vi "Dashboard Main.vi"() -> ()   [LabVIEW 2013]
uses:
  <vilib>/event_ctls.llb/eventvkey.ctl
  <vilib>/Rock Robotics/WPI/Dashboard/WPI_DashboardLogging Global.vi
  <vilib>/Utility/config.llb/Write Key (String).vi
  <vilib>/Utility/config.llb/Write Key (I32).vi
  <vilib>/Utility/config.llb/NI_LVConfig.lvlib
panel:
  out "Image Message":string="Timeout in Camera Communications"
  in  "Rec Mode":enum32{"Stop", "Record", "Playback"}(radio)
  in  "Dashboard Tab":T1(tab)
  in  "Camera Settings":T2={"Frame Rate"=30, "Compression"=30, "Size"=1} {"Frame Rate" scale=1.0..30.0; "Size" items=["640x480", "320x240", "160x120"]}
  out "MotorSliders R":cluster{"MotorSlide1":dbl, "MotorSlide2":dbl} {"MotorSlide2" scale=-1.0..1.0 scale format="%#_2e"; "MotorSlide1" scale=-1.0..1.0 scale format="%#_2e"}
  out "MotorChart R":cluster{"Numeric":dbl, "Numeric":dbl}(graph)
  out "MotorSliders L":T3 {"MotorSlide4 2" scale=0.0..14.0 scale format="%#_2e"; "MotorSlide2" scale=-1.0..1.0 scale format="%#_2e"; "MotorSlide1" scale=-1.0..1.0 scale format="%#_2e"}
  out "MotorChart L":T4(graph)
  out "JS1 Z":dbl(slide) scale=-1.0..1.0 scale format="%#_2e"
  out "Joystick 1":cluster{"X":dbl, "Y":dbl}[](graph)
  out "JS Buttons 1":T5
  out "JS2 Z":dbl(slide) scale=-1.0..1.0 scale format="%#_2e"
  out "Joystick 2":cluster{"X":dbl, "Y":dbl}[](graph)
  out "JS Buttons 2":T5
  out "Mode":T6(ring)=enum."Auto Disabled"
  out "Camera IP":string
  in  "DB Camera Config":bool
  out "fps":dbl format="%#.1g"
  out "Mbps":dbl format="%#.1g"
  out "Mbps 2":bool
  out "LED 1":bool
  in  "Experimental Features":bool
  in  "Camera Light":bool
  out "Shot Duration":dbl
  out "Shooting":bool
  in  "Fake LS":bool
  out "Light":dbl
  in  "Zero Encoders":bool
  out "Right Encoder":dbl
  out "Left Encoder":dbl
  out "Ultrasonic":dbl(slide) scale=0.0..14.0
  out "Pickup Solenoid Reverse":bool
  out "Pickup Solenoid Forward":bool
  out "Shooter Solenoid":bool
  out "Robot Code Version":string
  in  "Auto Routine":dbl
  in  "Shoot Distance":dbl
  in  "Distance from Tape":dbl
  out "Vision Display":T7(plugin-control)
  in  "Vision Processing":bool
  in  "Annotation":bool=TRUE
  in  "Retroreflective Processing":bool=TRUE
  in  "Team Color Processing":bool=TRUE
  out "Number of Particles":i32
  in  "Threshold Values":T8(array[cluster])
  in  "Introduce Photo":bool
  in  "Picture Input":path
  in  "Test Slider":dbl(slide) scale=0.0..100.0 scale format="%#_3g"
  in  "On/Off":bool caption="Solenoid"
  in  "Test Name":u16(ring) items=["Select the test to run...", "Example Test", "-------------------------------", "List of tests is built in robot code.", "Replace with your own automated tests."]
  in  "Test Tree":string(tree)
  in  "Motor":cluster{"Value":dbl, "Enable":bool} {"Value" scale=-1.0..1.0 scale format="%#_3g"}
  out "Progress":T9 {"Test Progress" scale=0.0..100.0}
  in  "Rev/Fwd":cluster{"Forward":bool, "Reverse":bool}
  in  "Test Ring":u16(ring) items=["Auto", "Fixed indoor", "Fixed outdoor 1", "Fixed outdoor 2", "Fixed fluorescent 1", "Fixed fluorescent 2", "Hold current"]
  in  "Listbox":i32(listbox)
  out "Tree":string(tree)
  out "Camera Image":T7(plugin-control)
  in  "Enable":bool
  # "Left"
  # "Front"
  # "Right"
  # "Battery"
  # "Set to 0 for none\nSet to 1 for Auto 1"
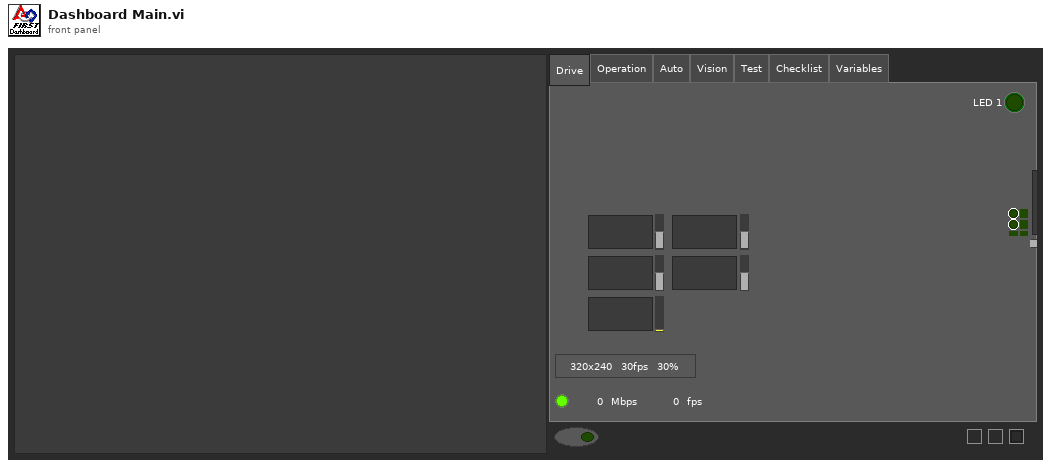
[diagram p1: front panel]
types:
  T1 = enum32{"Drive", "Operation", "Auto", "Vision", "Test", "Checklist", "Variables"}
  T2 = cluster{"Frame Rate":i32, "Compression":i32, "Size":u16}
  T3 = cluster{"MotorSlide1":dbl, "MotorSlide2":dbl, "MotorSlide4 2":dbl}
  T4 = cluster{"Numeric":dbl, "Numeric":dbl, "Battery":sgl}
  T5 = cluster{bool, bool, bool, bool, bool, bool, bool, bool, bool, bool, bool, bool}
  T6 = enum8{"Tele-Op Disabled", "Tele-Op Enabled", "Auto Disabled", "Auto Enabled", "Test Disabled", "Test Enabled", ""}
  T7 = typedef "IMAQ Image.ctl" = refnum<image>
  T8 = cluster{"Blue or Luma or Val or Inten Range":cluster{"Lower value":i32, "Upper value":i32}, "Red or Hue Range":cluster{"Lower value":i32, "Upper value":i32}, "Green or Sat Range":cluster{"Lower value":i32, "Upper value":i32}}[]
  T9 = cluster{"Test Progress":u8, "Test Progress Text":string}
  T10 = enum32{"Drive", "Operation", "Auto", "Test", "Checklist", "Variables"}
  T11 = typedef "Image Type" = u32
  T12 = cluster{"Digital Inputs":bool[], "Digital Outputs":bool[]}
  T13 = cluster{"Competition mode":bool, "Robot Link":bool, "Autonomous":bool, "Enabled":bool, "E-Stop":bool, "Simulated":bool, "TestMode":bool, "Docked Window":bool}
  T14 = cluster{"Boolean Array[0]":bool, "Boolean Array[1]":bool, "Boolean Array[2]":bool, "Boolean Array[3]":bool, "Boolean Array[4]":bool, "Boolean Array[5]":bool, "Boolean Array[6]":bool, "Boolean Array[7]":bool, "Boolean Array[8]":bool, "Boolean Array[9]":bool, "Boolean Array[10]":bool, "Boolean Array[11]":bool}
  T15 = typedef "NI_LVConfig.lvlib/Config Data RefNum.ctl" = refnum<k1>
  T16 = typedef "eventvkey.ctl" = enum16{"ASCII", "Enter", "Return", "Shift", "Ctrl", "Alt", "Cmd", "Opt", "Caps", "NumLock", "Clear", "Break", "Up", "Down", "Left", "Right", "Insert", "Delete", "Home", "End", "PageUp", "PageDown", "Escape", "Help", "Pause", "ScrollLock", "F1", "F2", "F3", "F4", "F5", "F6", "F7", "F8", "F9", "F10", "F11", "F12", "F13", "F14", "F15", "F16", "F17", "F18", "F19", "F20", "F21", "F22", "F23", "F24", "Play", "VolumeUp", "VolumeDown", "Mute", "Two Byte Char"}
  T17 = cluster{"Image Size":bool, "Image Type":bool, "Pixel Value":bool, "ROI Information":bool, "Zoom Factor":bool}
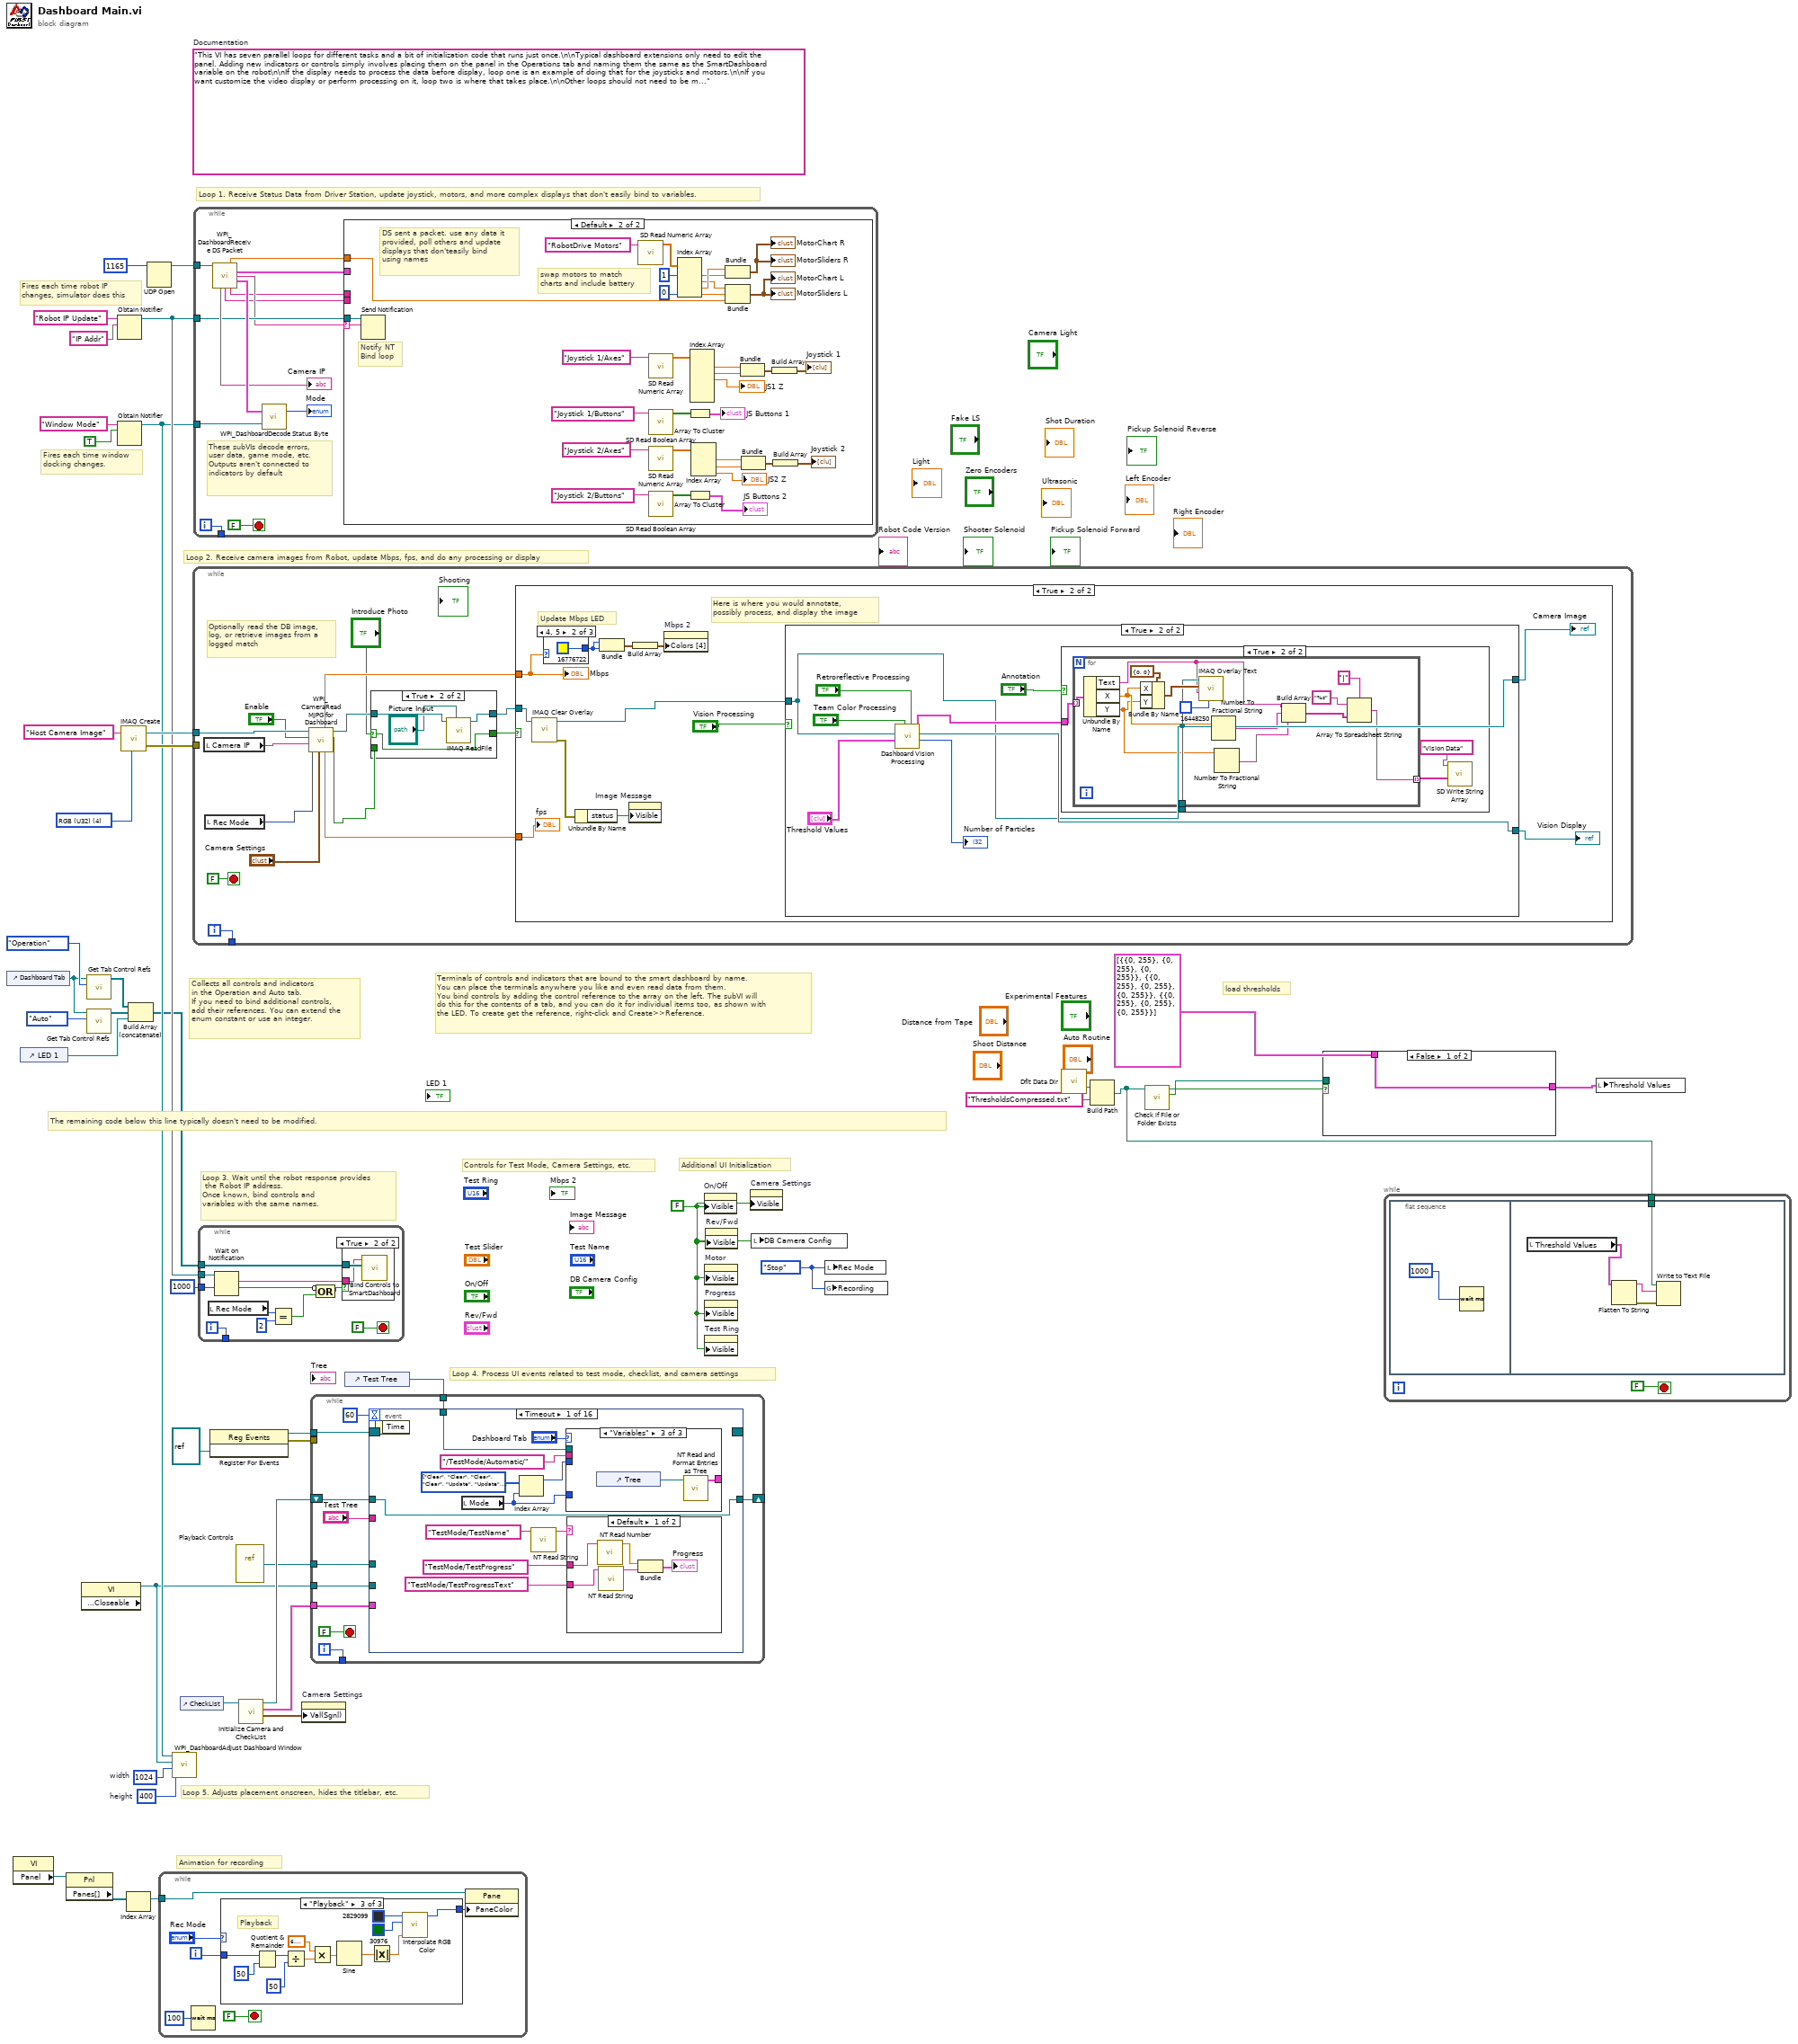
[diagram p0: block diagram]
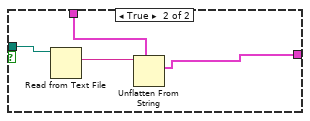
[diagram p2: hidden frame]
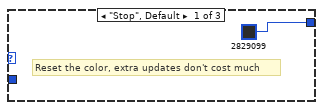
[diagram p3: hidden frame]
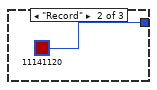
[diagram p4: hidden frame]
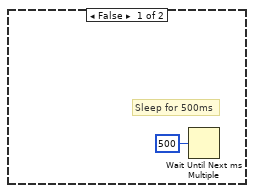
[diagram p7: hidden frame]
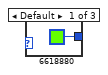
[diagram p10: hidden frame]
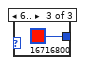
[diagram p11: hidden frame]
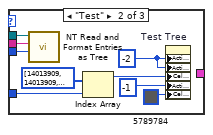
[diagram p13: hidden frame]
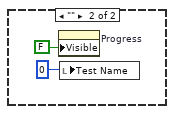
[diagram p14: hidden frame]
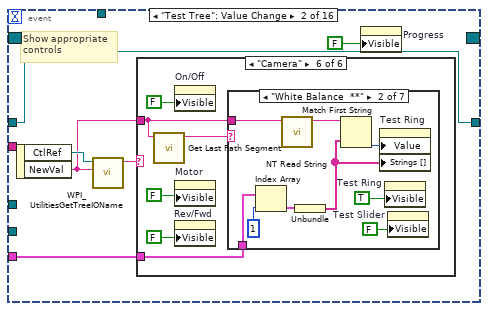
[diagram p15: hidden frame]
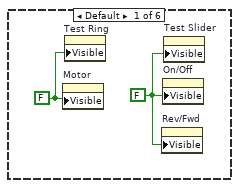
[diagram p16: hidden frame]
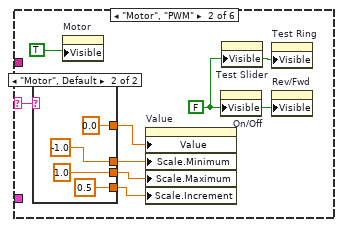
[diagram p17: hidden frame]
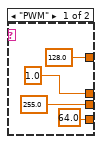
[diagram p18: hidden frame]
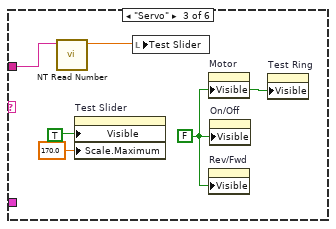
[diagram p19: hidden frame]
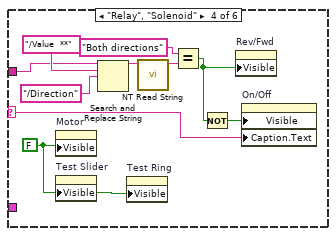
[diagram p20: hidden frame]
diagram:
  w15 = enum32{"Stop", "Record", "Playback"}."Stop" ("Rec Mode")
  w18 = 400  # height
  w19 = 1024  # width
  w32 = FALSE ("Visible")
  (unwired) "This VI has seven parallel loops for different tasks and a bit of initialization code that runs just once.\n\nTypical dashboard extensions only need to edit the panel. Adding new indicators or controls simply involves placing them on the panel in the Operations tab and naming them the same as the SmartDashboard variable on the robot\n\nIf the display needs to process the data before display, loop one is an example of doing that for the joysticks and motors.\n\nIf you want customize the video display or perform processing on it, loop two is where that takes place.\n\nOther loops should not need to be modified. They are pretty standard, and document the task they perform."  # Documentation
  w42 = T11 4 items=["Grayscale (U8)", "Grayscale (I16)", "Grayscale (SGL)", "Complex (CSG)", "RGB (U32)", "HSL (U32)", "RGB (U64)"] ("Image Type")
  # "load thresholds"
  # "Controls for Test Mode, Camera Settings, etc."
  # "Additional UI Initialization"
  # "Animation for recording"
  # "Fires each time robot IP\nchanges, simulator does this"
  # "Fires each time window\ndocking changes."
  # "Collects all controls and indicators\nin the Operation and Auto tab.\nIf you need to bind additional controls,\nadd their references. You can extend the\nenum constant or use an integer."
  # "The remaining code below this line typically doesn't need to be modified."
  # "Loop 4. Process UI events related to test mode, checklist, and camera settings"
  # "Terminals of controls and indicators that are bound to the smart dashboard by name.\nYou can place the terminals anywhere you like and even read data from them.\nYou bind controls by adding the control reference to the array on the left. The subVI will\ndo this for the contents of a tab, and you can do it for individual items too, as shown with\nthe LED. To create get the reference, right-click and Create>>Reference."
  # "Loop 3. Wait until the robot response provides\n the Robot IP address.\nOnce known, bind controls and\nvariables with the same names."
  # "Loop 5. Adjusts placement onscreen, hides the titlebar, etc."
  # "Loop 1. Receive Status Data from Driver Station, update joystick, motors, and more complex displays that don't easily bind to variables."
  # "Loop 2. Receive camera images from Robot, update Mbps, fps, and do any processing or display"
  n1 = control-ref of="Dashboard Tab"() -> (w13:refnum<vi>)
  n2 = property class="VI"() -> ("Panel"=w26:refnum<vi>)  [unwired: 2 in, 2 out]
  n3 = control-ref of="LED 1"() -> (w8:refnum<vi>)
  n4 = property class="Pnl"(reference=w26) -> ("Panes[]"=w27:refnum<vi>[])  [unwired: 1 in, 2 out]
  n5 = property class="VI" props=["Front Panel.Closeable"]() -> (reference out=w14:refnum<vi>)  [unwired: 2 in, 2 out]
  n6 = call <vilib>:"Get Tab Control Refs.vi"("Page Index"=T10."Operation" ("Dashboard Tab"), "TabControl in"=w13) -> ("ControlsOnPage"=w11:refnum<vi>[])  [unwired: 9 in]
  n7 = call <vilib>:"Get Tab Control Refs.vi"("Page Index"=T10."Auto" ("Dashboard Tab"), "TabControl in"=w13) -> ("ControlsOnPage"=w12:refnum<vi>[])  [unwired: 9 in]
  n8 = Obtain Notifier(name (unnamed)="Robot IP Update", notification data type="IP Addr" ("name (unnamed)")) -> (notifier out=w36:refnum<notifier>)  [unwired: 2 in, 2 out]
  n9 = Obtain Notifier(name (unnamed)="Window Mode", notification data type=TRUE) -> (notifier out=w17:refnum<notifier>)  [unwired: 2 in, 2 out]
  n10 = call "IMAQ Create"("Image Name"="Host Camera Image", "Image Type"=w42) -> ("New Image"=w40:T7, "error out"=w39:errorcluster)  [unwired: 2 in, 1 out]
  n11 = Index Array(array=w27) -> (element=w25:refnum<vi>)  [unwired: 1 in]
  n12 = Build Array (concatenate)(w11, w12, w8) -> (w10:refnum<vi>[])
  n13 = UDP Open(11:u16 1165 ("port")) -> (port=w43:refnum<k16>)  [unwired: 2 in, 4 out]
  n14 = while {
    tunnel: w25 -> [w46]
    i -> [w49]
    stop <- FALSE stop-if-true
    n15 = Wait (ms)(milliseconds to wait=u32 100) -> ()  [unwired: 1 out]
    n16 = case shown="\"Playback\"" "Rec Mode" {
      tunnel: w49 -> [_ _ w64]
      tunnel: [u32 2829099 ("Base Color") u32 11141120 ("Target Color") w53] -> w45
      frame "Stop", Default {
        # "Reset the color, extra updates don't cost much"
      }
      frame "Record" {
      }
      frame "Playback" {
        # "Playback"
        n17 = Quotient & Remainder(x=w64, y=u32 50 ("milliseconds to wait")) -> (x-y*floor(x/y)=w60:u32)  [unwired: 1 out]
        n18 = Divide(x=w60, y=u32 50 ("milliseconds to wait")) -> (x/y=w57:dbl)
        n19 = Multiply(x=6.283185307179586, y=w57) -> (x*y=w62:dbl)
        n20 = Sine(x=w62) -> (sin(x)=w61:dbl)
        n21 = Absolute Value(x=w61) -> (abs(x)=w54:dbl)
        n22 = call "Interpolate RGB Color.vi"("Proportion"=w54, "Target Color"=u32 30976, "Base Color"=u32 2829099) -> ("Result Color"=w53:u32)  [unwired: 8 in]
      }
    }
    n23 = property class="Pane"(reference=w46, "PaneColor"=w45) -> ()  [unwired: 1 in, 2 out]
  }
  n24 = call <vilib>:"WPI_DashboardAdjust Dashboard Window.vi"("height"=w18, "width"=w19, "reference in"=w14, "Notifier in"=w17) -> ()  [unwired: 8 in]
  n25 = control-ref of="CheckList"() -> (w16:refnum<vi>)
  n26 = while {
    tunnel: w40 -> [w76]
    tunnel: w39 -> [_]
    tunnel: [w77] -> _
    i -> [w77]
    stop <- FALSE stop-if-true
    # "Optionally read the DB image,\nlog, or retrieve images from a\nlogged match"
    n27 = local read "Camera IP"() -> (w71:string)
    n28 = local read "Rec Mode"() -> (w70:enum32{"Stop", "Record", "Playback"})
    n29 = call <vilib>:"WPI_CameraRead MJPG for Dashboard.vi"("Camera Settings"="Camera Settings", "Rec Mode"=w70, "Camera IP"=w71, "Enable"="Enable", "Refnum in"=w76) -> ("Active"=w66:bool, "Refnum out"=w69:T7, "FPS"=w74:dbl, "Bandwidth (Mbps)"=w73:dbl)  [unwired: 3 in]
    n30 = case shown="True" "Introduce Photo" {
      selector: "Introduce Photo" -> [_ w81]
      tunnel: w69 -> [w80 w84]
      tunnel: [w80 w83] -> w68
      tunnel: w66 -> [w79 _]
      tunnel: [w79 w81] -> w65
      frame False {
      }
      frame True {
        n31 = call "IMAQ ReadFile"("File Path"="Picture Input", "Image"=w84) -> ("Image Out"=w83:T7)  [unwired: 5 in, 4 out]
      }
    }
    n32 = case shown="True" w65 {
      tunnel: w73 -> [_ w92]
      tunnel: w74 -> [_ w91]
      tunnel: w68 -> [_ w87]
      frame False {
        # "Sleep for 500ms"
        n33 = Wait Until Next ms Multiple(millisecond multiple=u32 500) -> ()  [unwired: 1 out]
      }
      frame True {
        # "Here is where you would annotate,\npossibly process, and display the image"
        # "Update Mbps LED"
        n34 = call "IMAQ Clear Overlay"("Image"=w87) -> ("error out"=w96:errorcluster, "Image Out"=w89:T7)  [unwired: 2 in, 7 out]
        n35 = case shown="4, 5" w92 {
          tunnel: [u32 6618880 ("Color Box") u32 16776722 ("Color Box") u32 16716800 ("Color Box")] -> w93
          frame Default {
          }
          frame 4, 5 {
          }
          frame 6.. {
          }
        }
        n36 = Unbundle By Name(w96) -> ("status"=w97:bool)
        n37 = Bundle("Color Box"=w93, "Color Box"=w93) -> (w95:cluster{"Color Box":u32, "Color Box":u32})  [unwired: 1 out]
        n38 = property on="Image Message" class="Str"("Visible"=w97) -> ()  [unwired: 2 in, 2 out]
        n39 = Build Array(w95) -> (w94:cluster{"Color Box":u32, "Color Box":u32}[])
        n40 = property on="Mbps 2" class="Bool (strict)"("Colors [4]"=w94) -> ()  [unwired: 2 in, 2 out]
        n41 = case shown="True" "Vision Processing" {
          tunnel: w89 -> [w98 w100]
          tunnel: [w98 w106] -> w86
          tunnel: [w98 w100] -> w88
          frame False {
          }
          frame True {
            n42 = call "Dashboard Vision Processing.vi"("Retroreflective Processing"="Retroreflective Processing", "Team Color Processing"="Team Color Processing", "Threshold Values"="Threshold Values", "Camera Image"=w100) -> ("Number of Particles"=→"Number of Particles":i32, "Retro Image"=w106:T7, "Annotations"=w101:cluster{"Text":string, "X":dbl, "Y":dbl}[])  [unwired: 4 in, 1 out]
            n43 = case shown="True" "Annotation" {
              tunnel: w101 -> [_ w110]
              tunnel: w100 -> [_ w109]
              frame False {
              }
              frame True {
                n44 = for {
                  tunnel: w110 -> [w124] mode=indexing
                  tunnel: w109 -> [w121]
                  tunnel: [w111] -> w108 mode=indexing
                  n45 = Unbundle By Name(w124) -> ("Text"=w117:string, "X"=w120:dbl, "Y"=w119:dbl)
                  n46 = Bundle By Name(cluster=cluster{"X":i32, "Y":i32} {"X"=0, "Y"=0} ("Origin"), "X"=w120, "Y"=w119) -> (w122:cluster{"X":i32, "Y":i32})
                  n47 = call "IMAQ Overlay Text"("Text Color (black)"=u32 16448250, "String"=w117, "Origin"=w122, "Image"=w121) -> ()  [unwired: 6 in, 2 out]
                  n48 = Number To Fractional String(number=w120) -> (F-format string=w116:string)  [unwired: 3 in]
                  n49 = Number To Fractional String(number=w119) -> (F-format string=w115:string)  [unwired: 3 in]
                  n50 = Build Array(w117, w116, w115) -> (w114:string[])
                  n51 = Array To Spreadsheet String(delimiter (Tab)="|", array=w114, 3:"%s") -> (spreadsheet string=w111:string)
                }
                n52 = call <vilib>:"SD Write String Array.vi"("String Array"=w108, "Name"="Vision Data") -> ()  [unwired: 8 in, 2 out]
              }
            }
          }
        }
        "Camera Image" <- w88
        "Vision Display" <- w86
        "Mbps" <- w92
        "fps" <- w91
      }
    }
  }
  n53 = while {
    tunnel: w43 -> [w138]
    tunnel: w36 -> [w133]
    tunnel: w17 -> [w137]
    tunnel: [w134] -> _
    i -> [w134]
    stop <- FALSE stop-if-true
    # "These subVIs decode errors, user data, game mode, etc.\nOutputs aren't connected to indicators by default"
    n54 = call <vilib>:"WPI_DashboardReceive DS Packet.vi"("Recv Socket"=w138) -> ("Battery"=w128:sgl, "Driver Station"=w129:T12, "Robot IP Address"=w132:string, "Status"=w139:T13, "Camera IP Address"=→"Camera IP":string, "Low Priority User Data"=w131:string, "High Priority User Data"=w130:string)  [unwired: 1 in, 7 out]
    n55 = call <vilib>:"WPI_DashboardDecode Status Byte.vi"("Window Mode Notifier"=w137, "Status"=w139) -> ("Mode"=→"Mode":T6)  [unwired: 1 out]
    n56 = case shown="Default" w132 {
      selector: w132 -> [_ w151]
      tunnel: w133 -> [_ w152]
      tunnel: w131 -> [_ _]
      tunnel: w130 -> [_ _]
      tunnel: w129 -> [_ _]
      tunnel: w128 -> [_ w150]
      frame "0.0.0.0" {
        # "DS not sending packets, or no robot exists yet.\nDon't poll the variables"
      }
      frame Default {
        # "Notify NT\nBind loop"
        # "DS sent a packet. use any data it\nprovided, poll others and update\ndisplays that don'teasily bind\nusing names"
        # "swap motors to match\ncharts and include battery"
        n57 = Send Notification(notification=w151, notifier=w152) -> ()  [unwired: 1 in, 2 out]
        n58 = call <vilib>:"SD Read Numeric Array.vi"("Name"="RobotDrive Motors") -> ("Numeric Array"=w149:dbl[])  [unwired: 8 in, 2 out]
        n59 = call <vilib>:"SD Read Numeric Array.vi"("Name"="Joystick 1/Axes") -> ("Numeric Array"=w168:dbl[])  [unwired: 8 in, 2 out]
        n60 = call <vilib>:"SD Read Boolean Array.vi"("Name"="Joystick 1/Buttons") -> ("Boolean Array"=w170:bool[])  [unwired: 8 in, 2 out]
        n61 = call <vilib>:"SD Read Numeric Array.vi"("Name"="Joystick 2/Axes") -> ("Numeric Array"=w162:dbl[])  [unwired: 8 in, 2 out]
        n62 = call <vilib>:"SD Read Boolean Array.vi"("Name"="Joystick 2/Buttons") -> ("Boolean Array"=w161:bool[])  [unwired: 8 in, 2 out]
        n63 = Index Array(array=w149, index #1=1, index #4=0) -> (element #1=w145:dbl, element #2=w144:dbl, element #3=w146:dbl, element #4=w141:dbl)  [unwired: 2 in]
        n64 = Array To Cluster(array=w170) -> (cluster=→"JS Buttons 1":T14)
        n65 = Array To Cluster(array=w161) -> (cluster=→"JS Buttons 2":T14)
        n66 = Index Array(array=w168) -> (element #1=w165:dbl, element #2=w166:dbl, element #3=→"JS1 Z":dbl)  [unwired: 6 in, 3 out]
        n67 = Index Array(array=w162) -> (element #1=w157:dbl, element #2=w156:dbl, element #3=→"JS2 Z":dbl)  [unwired: 3 in]
        n68 = Bundle("Numeric"=w146, "Numeric"=w145) -> (→"MotorChart R" →"MotorSliders R":cluster{"Numeric":dbl, "Numeric":dbl})  [unwired: 1 in]
        n69 = Bundle("Numeric"=w144, "Numeric"=w141, "Battery"=w150) -> (→"MotorChart L" →"MotorSliders L":T4)  [unwired: 1 in]
        n70 = Bundle("Numeric"=w165, "Numeric"=w166) -> (w164:cluster{"Numeric":dbl, "Numeric":dbl})  [unwired: 1 in]
        n71 = Bundle("Numeric"=w157, "Numeric"=w156) -> (w158:cluster{"Numeric":dbl, "Numeric":dbl})  [unwired: 1 in]
        n72 = Build Array(w164) -> (→"Joystick 1":cluster{"Numeric":dbl, "Numeric":dbl}[])
        n73 = Build Array(w158) -> (→"Joystick 2":cluster{"Numeric":dbl, "Numeric":dbl}[])
      }
    }
  }
  n74 = while {
    tunnel: w10 -> [w184]
    tunnel: w36 -> [w182]
    tunnel: [w180] -> _
    tunnel: u32 1000 ("milliseconds to wait") -> [w179]
    i -> [w180]
    stop <- FALSE stop-if-true
    n75 = local read "Rec Mode"() -> (w175:enum32{"Stop", "Record", "Playback"})
    n76 = Wait on Notification(notifier=w182, timeout in ms (-1)=w179) -> (notification=w181:string, timed out?=w177:bool)  [unwired: 2 in, 2 out]
    n77 = Equal?(x=w175, y=u16 2 ("Rec Mode")) -> (x = y?=w176:bool)
    n78 = Compound Arithmetic op=OR(invert w177, w176) -> (w178:bool)
    n79 = case shown="True" w178 {
      tunnel: w184 -> [_ w186]
      tunnel: w181 -> [_ w185]
      frame False {
      }
      frame True {
        n80 = call <vilib>:"Bind Controls to SmartDashboard.vi"("Bound Control Refs"=w186, "Server IP Address"=w185) -> ()  [unwired: 10 in]
      }
    }
  }
  n81 = register-events(refnum<vi> refnum) -> (reference out=w23:refnum<event-registration>, error out=w22:errorcluster)  [unwired: 2 in]
  n82 = vi-ref "Playback Controls.vi"() -> (w24:refnum<vi>)
  n83 = call "Initialize Camera and CheckList.vi"("ListBox in"=w16) -> ("Cluster"=w30:cluster{"value":i32, "value":i32, "index":i32}, "Array"=w31:cluster{string[]}[], "File Refnum"=w29:T15)  [unwired: 8 in]
  n84 = property on="Camera Settings" class="Clust (strict)"("Val(Sgnl)"=w30) -> ()  [unwired: 2 in, 2 out]
  n85 = control-ref of="Test Tree"() -> (w28:refnum<vi>)
  n86 = while {
    tunnel: w31 -> [w194]
    shift-right: [w193] -> _
    shift-left: w29 -> [w192]
    tunnel: [w191] -> _
    tunnel: w28 -> [w190]
    tunnel: w24 -> [w189]
    tunnel: w23 -> [w188]
    tunnel: w22 -> [_]
    tunnel: w14 -> [w187]
    i -> [w191]
    stop <- FALSE stop-if-true
    n87 = event shown="[0] Timeout" {
      selector: w188 -> [_ _ _ _ _ _ _ _ _ _ _ _ _ _ _ _]
      dyn-events: [_ _ _ _ _ _ _ _ _ _ _ _ _ w432 _ _] -> _
      timeout: u32 60 ("milliseconds to wait") -> [_ _ _ _ _ _ _ _ _ _ _ _ _ _ _ _]
      tunnel: w190 -> [w204 _ _ _ _ _ _ _ _ _ _ _ _ _ _ _]
      tunnel: "Test Tree" -> [_ _ _ _ _ _ _ _ w401 w409 w411 w415 w423 _ _ _]
      tunnel: w194 -> [_ w228 _ _ _ _ w365 w395 _ _ _ _ _ _ _ _]
      tunnel: [w198 w227 w326 w331 w339 w351 w364 w388 w400 w407 w410 w414 w422 w434 w448 w449] -> w193
      tunnel: w192 -> [w198 w227 w326 w331 w339 w351 w363 w388 w400 w407 w410 w414 w422 w434 w448 w449]
      tunnel: w189 -> [_ _ _ _ _ _ _ _ _ _ _ _ _ w435 _ w452]
      tunnel: w187 -> [_ _ _ _ _ _ _ _ _ _ _ _ _ w430 _ _]
      event Timeout {
        w203 = enum16{"Update", "Clear"}[] [enum."Clear", enum."Clear", enum."Clear", enum."Clear", enum."Update", enum."Update", enum."Clear"] items=["Update", "Clear"]
        n88 = event-data() -> ()  [unwired: 1 in, 1 out]
        n89 = local read "Mode"() -> (w201:T6)
        n90 = Index Array(array=w203, index=w201) -> (element=w202:enum16{"Update", "Clear"})
        n91 = call <vilib>:"NT Read String.vi"("Name"="TestMode/TestName") -> ("String"=w207:string)  [unwired: 9 in, 1 out]
        n92 = case shown="\"Variables\"" "Dashboard Tab" {
          tunnel: w204 -> [_ w217 _]
          tunnel: "/TestMode/Automatic/" ("Name Pattern") -> [_ w216 _]
          tunnel: w202 -> [_ w215 _]
          tunnel: w201 -> [_ w213 _]
          tunnel: [_ _ w219] -> _
          frame "Operation", Default {
          }
          frame "Test" {
            w212 = -2 ("Active Item:Row Number")
            n93 = call <vilib>:"NT Read and Format Entries as Tree.vi"("Operation"=w215, "Name Pattern"=w216, "Tree Refnum"=w217) -> ()  [unwired: 7 in, 2 out]
            n94 = Index Array(array=u32[] [14013909, 14013909, 14013909, 14013909, 14013909, 16777215, 14013909], index=w213) -> (element=w211:u32)
            n95 = property on="Test Tree" class="Tree (strict)"("Active Item Row Number"=w212, "ActiveColNum"=w212, "CellBG"=w211, "Active Item Row Number"=-1 ("Active Item:Row Number"), "CellBG"=u32 5789784 ("Color Box")) -> ()  [unwired: 2 in, 2 out]
          }
          frame "Variables" {
            n96 = control-ref of="Tree"() -> (w218:refnum<vi>)
            n97 = call <vilib>:"NT Read and Format Entries as Tree.vi"("Tree Refnum"=w218) -> ("Formatted Strings"=w219:cluster{"Name":string, "Value":string}[])  [unwired: 9 in, 1 out]
          }
        }
        n98 = case shown="Default" w207 {
          tunnel: "TestMode/TestProgress" ("Name") -> [w221 _]
          tunnel: "TestMode/TestProgressText" ("Name") -> [w220 _]
          frame Default {
            n99 = call <vilib>:"NT Read Number.vi"("Name"=w221) -> ("Numeric"=w222:dbl)  [unwired: 9 in, 1 out]
            n100 = call <vilib>:"NT Read String.vi"("Name"=w220) -> ("String"=w223:string)  [unwired: 9 in, 1 out]
            n101 = Bundle("Numeric"=w222, "String"=w223) -> (→"Progress":cluster{"Numeric":dbl, "String":string})  [unwired: 1 in]
          }
          frame "" {
            n102 = property on="Progress" class="Clust (strict)"("Visible"=FALSE) -> ()  [unwired: 2 in, 2 out]
            n103 = local write "Test Name"(u16 0) -> ()
          }
        }
      }
      event "Test Tree": Value Change {
        # "Show appropriate\ncontrols"
        n104 = event-data() -> ("CtlRef"=w231:refnum<vi>, "NewVal"=w229:string)  [unwired: 1 in]
        n105 = call <vilib>:"WPI_UtilitiesGetTreeIOName.vi"("NewVal"=w229, "TreeControl in"=w231) -> ("I/O Name"=w232:string)  [unwired: 9 in]
        n106 = case shown="\"Camera\"" w232 {
          selector: w232 -> [_ w239 _ w257 w266 _]
          tunnel: w229 -> [_ _ w254 w256 _ w273]
          tunnel: w228 -> [_ _ _ _ _ w272]
          frame Default {
            w234 = FALSE ("Visible")
            w233 = FALSE ("Visible")
            n107 = property on="Motor" class="Clust (strict)"("Visible"=w233) -> ()  [unwired: 2 in, 2 out]
            n108 = property on="Test Ring" class="Ring (strict)"("Visible"=w233) -> ()  [unwired: 2 in, 2 out]
            n109 = property on="Rev/Fwd" class="Clust (strict)"("Visible"=w234) -> ()  [unwired: 2 in, 2 out]
            n110 = property on="On/Off" class="Bool (strict)"("Visible"=w234) -> ()  [unwired: 2 in, 2 out]
            n111 = property on="Test Slider" class="Slide (strict)"("Visible"=w234) -> ()  [unwired: 2 in, 2 out]
          }
          frame "Motor", "PWM" {
            w240 = FALSE ("Visible")
            n112 = case shown="\"Motor\", Default" w239 {
              tunnel: [1.0 ("Value") -1.0 ("Value")] -> w238
              tunnel: [255.0 ("Value") 1.0 ("Value")] -> w237
              tunnel: [128.0 ("Value") 0.0 ("Value")] -> w236
              tunnel: [64.0 ("Value") 0.5 ("Value")] -> w235
              frame "PWM" {
              }
              frame "Motor", Default {
              }
            }
            n113 = property on="Motor" class="Clust (strict)"("Visible"=TRUE) -> ()  [unwired: 2 in, 2 out]
            n114 = property on="Value" class="Slide (strict)"("Value"=w236, "Scale.Minimum"=w238, "Scale.Maximum"=w237, "Scale.Increment"=w235) -> ()  [unwired: 2 in, 2 out]
            n115 = property on="On/Off" class="Bool (strict)"("Visible"=w240) -> ()  [unwired: 2 in, 2 out]
            n116 = property on="Test Slider" class="Slide (strict)"("Visible"=w240) -> ()  [unwired: 2 in, 2 out]
            n117 = property on="Test Ring" class="Ring (strict)"("Visible"=w240) -> ()  [unwired: 2 in, 2 out]
            n118 = property on="Rev/Fwd" class="Clust (strict)"("Visible"=w240) -> ()  [unwired: 2 in, 2 out]
          }
          frame "Servo" {
            w252 = FALSE ("Visible")
            n119 = call <vilib>:"NT Read Number.vi"("Name"=w254) -> ("Numeric"=w253:dbl)  [unwired: 9 in, 1 out]
            n120 = property on="Test Slider" class="Slide (strict)"("Visible"=TRUE, "Scale.Maximum"=170.0 ("Scale.Range:Maximum")) -> ()  [unwired: 2 in, 2 out]
            n121 = local write "Test Slider"(w253) -> ()
            n122 = property on="Motor" class="Clust (strict)"("Visible"=w252) -> ()  [unwired: 2 in, 2 out]
            n123 = property on="Rev/Fwd" class="Clust (strict)"("Visible"=w252) -> ()  [unwired: 2 in, 2 out]
            n124 = property on="On/Off" class="Bool (strict)"("Visible"=w252) -> ()  [unwired: 2 in, 2 out]
            n125 = property on="Test Ring" class="Ring (strict)"("Visible"=w252) -> ()  [unwired: 2 in, 2 out]
          }
          frame "Relay", "Solenoid" {
            w255 = FALSE ("Visible")
            n126 = property on="Motor" class="Clust (strict)"("Visible"=w255) -> ()  [unwired: 2 in, 2 out]
            n127 = property on="Test Slider" class="Slide (strict)"("Visible"=w255) -> ()  [unwired: 2 in, 2 out]
            n128 = Search and Replace String(input string=w256, search string="/Value  **", replace string="/Direction") -> (result string=w262:string)  [unwired: 5 in, 3 out]
            n129 = property on="Test Ring" class="Ring (strict)"("Visible"=w255) -> ()  [unwired: 2 in, 2 out]
            n130 = call <vilib>:"NT Read String.vi"("Name"=w262) -> ("String"=w260:string)  [unwired: 9 in, 1 out]
            n131 = Equal?(x="Both directions", y=w260) -> (x = y?=w258:bool)
            n132 = Not(x=w258) -> (.not. x?=w259:bool)
            n133 = property on="Rev/Fwd" class="Clust (strict)"("Visible"=w258) -> ()  [unwired: 2 in, 2 out]
            n134 = property on="On/Off" class="Bool (strict)"("Visible"=w259, "Caption.Text"=w257) -> ()  [unwired: 2 in, 2 out]
          }
          frame "Compressor", "Digital Out" {
            w265 = FALSE ("Visible")
            # "Get direction and finish"
            n135 = property on="Motor" class="Clust (strict)"("Visible"=w265) -> ()  [unwired: 2 in, 2 out]
            n136 = property on="Test Slider" class="Slide (strict)"("Visible"=w265) -> ()  [unwired: 2 in, 2 out]
            n137 = property on="Test Ring" class="Ring (strict)"("Visible"=w265) -> ()  [unwired: 2 in, 2 out]
            n138 = property on="On/Off" class="Bool (strict)"("Visible"=TRUE, "Caption.Text"=w266) -> ()  [unwired: 2 in, 2 out]
            n139 = property on="Rev/Fwd" class="Clust (strict)"("Visible"=FALSE) -> ()  [unwired: 2 in, 2 out]
          }
          frame "Camera" {
            n140 = call <vilib>:"Get Last Path Segment.vi"("String in"=w273) -> ("String out"=w274:string)  [unwired: 10 in]
            n141 = property on="On/Off" class="Bool (strict)"("Visible"=FALSE) -> ()  [unwired: 2 in, 2 out]
            n142 = property on="Motor" class="Clust (strict)"("Visible"=FALSE) -> ()  [unwired: 2 in, 2 out]
            n143 = property on="Rev/Fwd" class="Clust (strict)"("Visible"=FALSE) -> ()  [unwired: 2 in, 2 out]
            n144 = case shown="\"White Balance  **\"" w274 {
              tunnel: w273 -> [w280 w289 w298 w307 w316 _ w322]
              tunnel: w272 -> [w278 w286 w295 w304 w313 _ _]
              frame "Size  **" {
                n145 = Index Array(array=w278) -> (element=w277:cluster{string[]})  [unwired: 1 in]
                n146 = call <vilib>:"NT Read String.vi"("Name"=w280) -> ("String"=w279:string)  [unwired: 9 in, 1 out]
                n147 = Unbundle(w277) -> (w275:string[])
                n148 = Match First String(2:w275, 3:w279) -> (0:w276:i32)  [unwired: 1 out]
                n149 = property on="Test Ring" class="Ring (strict)"("Value"=w276, "Strings []"=w275) -> ()  [unwired: 2 in, 2 out]
                n150 = property on="Test Ring" class="Ring (strict)"("Visible"=TRUE) -> ()  [unwired: 2 in, 2 out]
                n151 = property on="Test Slider" class="Slide (strict)"("Visible"=FALSE) -> ()  [unwired: 2 in, 2 out]
              }
              frame "White Balance  **" {
                n152 = Index Array(array=w286, index=1) -> (element=w287:cluster{string[]})
                n153 = call <vilib>:"NT Read String.vi"("Name"=w289) -> ("String"=w288:string)  [unwired: 9 in, 1 out]
                n154 = Unbundle(w287) -> (w284:string[])
                n155 = Match First String(2:w284, 3:w288) -> (0:w283:i32)  [unwired: 1 out]
                n156 = property on="Test Ring" class="Ring (strict)"("Value"=w283, "Strings []"=w284) -> ()  [unwired: 2 in, 2 out]
                n157 = property on="Test Ring" class="Ring (strict)"("Visible"=TRUE) -> ()  [unwired: 2 in, 2 out]
                n158 = property on="Test Slider" class="Slide (strict)"("Visible"=FALSE) -> ()  [unwired: 2 in, 2 out]
              }
              frame "Exposure  **" {
                n159 = Index Array(array=w295, index=2) -> (element=w296:cluster{string[]})
                n160 = call <vilib>:"NT Read String.vi"("Name"=w298) -> ("String"=w297:string)  [unwired: 9 in, 1 out]
                n161 = Unbundle(w296) -> (w292:string[])
                n162 = Match First String(2:w292, 3:w297) -> (0:w293:i32)  [unwired: 1 out]
                n163 = property on="Test Ring" class="Ring (strict)"("Value"=w293, "Strings []"=w292) -> ()  [unwired: 2 in, 2 out]
                n164 = property on="Test Ring" class="Ring (strict)"("Visible"=TRUE) -> ()  [unwired: 2 in, 2 out]
                n165 = property on="Test Slider" class="Slide (strict)"("Visible"=FALSE) -> ()  [unwired: 2 in, 2 out]
              }
              frame "Exposure Priority  **" {
                n166 = Index Array(array=w304, index=3) -> (element=w305:cluster{string[]})
                n167 = call <vilib>:"NT Read String.vi"("Name"=w307) -> ("String"=w306:string)  [unwired: 9 in, 1 out]
                n168 = Unbundle(w305) -> (w301:string[])
                n169 = Match First String(2:w301, 3:w306) -> (0:w302:i32)  [unwired: 1 out]
                n170 = property on="Test Ring" class="Ring (strict)"("Value"=w302, "Strings []"=w301) -> ()  [unwired: 2 in, 2 out]
                n171 = property on="Test Ring" class="Ring (strict)"("Visible"=TRUE) -> ()  [unwired: 2 in, 2 out]
                n172 = property on="Test Slider" class="Slide (strict)"("Visible"=FALSE) -> ()  [unwired: 2 in, 2 out]
              }
              frame "Color Enable  **" {
                n173 = Index Array(array=w313, index=4) -> (element=w314:cluster{string[]})
                n174 = call <vilib>:"NT Read String.vi"("Name"=w316) -> ("String"=w315:string)  [unwired: 9 in, 1 out]
                n175 = Unbundle(w314) -> (w310:string[])
                n176 = Match First String(2:w310, 3:w315) -> (0:w311:i32)  [unwired: 1 out]
                n177 = property on="Test Ring" class="Ring (strict)"("Value"=w311, "Strings []"=w310) -> ()  [unwired: 2 in, 2 out]
                n178 = property on="Test Ring" class="Ring (strict)"("Visible"=TRUE) -> ()  [unwired: 2 in, 2 out]
                n179 = property on="Test Slider" class="Slide (strict)"("Visible"=FALSE) -> ()  [unwired: 2 in, 2 out]
              }
              frame Default {
                n180 = property on="Test Ring" class="Ring (strict)"("Visible"=FALSE) -> ()  [unwired: 2 in, 2 out]
                n181 = property on="Test Slider" class="Slide (strict)"("Visible"=FALSE) -> ()  [unwired: 2 in, 2 out]
              }
              frame "Brightness  **", "Color Level  **", "Compression  **", "FPS  **", "Sharpness  **" {
                n182 = call <vilib>:"NT Read Number.vi"("Name"=w322) -> ("Numeric"=w321:dbl)  [unwired: 9 in, 1 out]
                n183 = local write "Test Slider"(w321) -> ()
                n184 = property on="Test Slider" class="Slide (strict)"("Visible"=TRUE, "Scale.Maximum"=100.0 ("Scale.Range:Maximum")) -> ()  [unwired: 2 in, 2 out]
                n185 = property on="Test Ring" class="Ring (strict)"("Visible"=FALSE) -> ()  [unwired: 2 in, 2 out]
              }
            }
          }
        }
        n186 = property on="Progress" class="Clust (strict)"("Visible"=FALSE) -> ()  [unwired: 2 in, 2 out]
      }
      event "Test Name": Mouse Enter {
        # "Populate the ring with the list of tests"
        n187 = event-data() -> ()  [unwired: 1 in, 1 out]
        n188 = call <vilib>:"NT Read String Array.vi"("Name"="TestMode/TestList") -> ("String Array"=w330:string[])  [unwired: 9 in, 1 out]
        n189 = Build Array (concatenate)("Select the test to run...", w330) -> (w329:string[])
        n190 = property on="Test Name" class="Ring (strict)"("Strings []"=w329) -> ()  [unwired: 2 in, 2 out]
      }
      event "Test Name": Value Change {
        w332 = FALSE ("Visible")
        # "Tell the robot the test name to run"
        n191 = event-data() -> ("NewVal"=w336:u16)  [unwired: 1 in]
        n192 = property on="Test Name" class="Ring (strict)"() -> ("Strings []"=w337:string[])  [unwired: 2 in, 2 out]
        n193 = local write "Progress"(T9 {"Test Progress"=0, "Test Progress Text"=""} ("Progress")) -> ()
        n194 = Index Array(array=w337, index=w336) -> (element=w335:string)
        n195 = call <vilib>:"NT Write String.vi"("String"=w335, "Name"="TestMode/TestName") -> ()  [unwired: 9 in, 1 out]
        n196 = property on="Progress" class="Clust (strict)"("Visible"=TRUE) -> ()  [unwired: 2 in, 2 out]
        n197 = property on="Motor" class="Clust (strict)"("Visible"=w332) -> ()  [unwired: 2 in, 2 out]
        n198 = property on="Test Slider" class="Slide (strict)"("Visible"=w332) -> ()  [unwired: 2 in, 2 out]
        n199 = property on="On/Off" class="Bool (strict)"("Visible"=w332) -> ()  [unwired: 2 in, 2 out]
        n200 = property on="Rev/Fwd" class="Clust (strict)"("Visible"=w332) -> ()  [unwired: 2 in, 2 out]
        n201 = property on="Test Ring" class="Ring (strict)"("Visible"=w332) -> ()  [unwired: 2 in, 2 out]
      }
      event "Listbox": Double Click {
        n202 = event-data() -> ("PlatMods.Shift"=w340:bool, "Row"=w342:i32)  [unwired: 1 in]
        n203 = case shown="True" w340 {
          tunnel: w342 -> [w346 _]
          tunnel: 1 -> [w345 _]
          frame False {
            n204 = property on="Listbox" class="LstBox (strict)"() -> ("Item Symbols"=w344:i32[])  [unwired: 2 in, 2 out]
            n205 = Replace Array Subset(array=w344, new element=w345, index=w346) -> (w343:i32[])
            n206 = property on="Listbox" class="LstBox (strict)"("Item Symbols"=w343) -> ()  [unwired: 2 in, 2 out]
          }
          frame True {
            w347 = 0 ("Top Row")
            n207 = property on="Listbox" class="LstBox (strict)"() -> ("Number of Rows"=w349:u32)  [unwired: 2 in, 2 out]
            n208 = Initialize Array(0, w349) -> (w348:i32[])
            n209 = property on="Listbox" class="LstBox (strict)"("Top Row"=w347, "Value"=w347, "Item Symbols"=w348) -> ()  [unwired: 2 in, 2 out]
          }
        }
      }
      event "Listbox": Key Down {
        n210 = event-data() -> ("VKey"=w353:T16)  [unwired: 1 in]
        n211 = case shown="\"Left\", \"Right\"" w353 {
          selector: w353 -> [w358 _]
          tunnel: eventvkey."Left" ("VKey") -> [w356 _]
          frame "Left", "Right" {
            n212 = Equal?(x=w356, y=w358) -> (x = y?=w357:bool)
            n213 = Select(t=0, s=w357, f=1) -> (s? t:f=w359:i32)
            n214 = property on="Listbox" class="LstBox (strict)"() -> ("Item Symbols"=w362:i32[])  [unwired: 2 in, 2 out]
            n215 = Replace Array Subset(array=w362, new element=w359, index="Listbox") -> (w361:i32[])
            n216 = property on="Listbox" class="LstBox (strict)"("Item Symbols"=w361) -> ()  [unwired: 2 in, 2 out]
          }
          frame Default {
          }
        }
      }
      event "DB Camera Config": Value Change {
        n217 = event-data() -> ("NewVal"=w366:bool)  [unwired: 1 in]
        n218 = case shown="False" w366 {
          tunnel: w365 -> [w375 _]
          tunnel: [w368 w386] -> w364
          tunnel: w363 -> [w367 w386]
          frame False {
            w382 = "Camera"
            w385 = FALSE ("Visible")
            n219 = local read "Camera Settings"() -> (w374:T2)
            n220 = Index Array(array=w375) -> (element=w378:cluster{string[]})  [unwired: 1 in]
            n221 = Unbundle(w374) -> ("Frame Rate"=w373:i32, "Compression"=w372:i32, "Size"=w376:u16)
            n222 = Unbundle(w378) -> (w377:string[])
            n223 = Index Array(array=w377, index=w376) -> (element=w371:string)
            n224 = call-poly <vilib>:"Write Key.vi"("section"=w382, "value"=w371, "key"="Size", "refnum"=w367) -> ("refnum out"=w384:T15)  [unwired: 2 in, 5 out]
            n225 = call-poly <vilib>:"Write Key.vi"("section"=w382, "value"=w373, "key"="FrameRate", "refnum"=w384) -> ("refnum out"=w383:T15)  [unwired: 1 in, 6 out]
            n226 = property on="Camera Settings" class="Clust (strict)"("Visible"=w385) -> ()  [unwired: 2 in, 2 out]
            n227 = local write "DB Camera Config"(w385) -> ()
            n228 = call-poly <vilib>:"Write Key.vi"("section"=w382, "value"=w372, "key"="Compression", "refnum"=w383) -> ("refnum out"=w369:T15)  [unwired: 1 in, 6 out]
            n229 = call <vilib>:"Close Config Data.vi"("refnum"=w369) -> ("file path"=w370:path)  [unwired: 2 in, 8 out]
            n230 = call <vilib>:"Open Config Data.vi"("configuration file path"=w370) -> ("refnum"=w368:T15)  [unwired: 8 in, 2 out]
          }
          frame True {
            n231 = property on="Camera Settings" class="Clust (strict)"("Visible"=TRUE) -> ()  [unwired: 2 in, 2 out]
          }
        }
      }
      event "Camera Settings": Value Change {
        n232 = event-data() -> ("NewVal"=w399:T2)  [unwired: 1 in]
        n233 = Index Array(array=w395) -> (element=w394:cluster{string[]})  [unwired: 1 in]
        n234 = Unbundle(w399) -> ("Frame Rate"=w390:i32, "Compression"=w389:i32, "Size"=w392:u16)
        n235 = Unbundle(w394) -> (w393:string[])
        n236 = Index Array(array=w393, index=w392) -> (element=w391:string)
        n237 = Format Into String(format string="%s   %dfps   %d%%", w391, w390, w389) -> (resulting string=w396:string)  [unwired: 2 in, 1 out]
        n238 = Build Array(w396) -> (w397:string[])
        n239 = property on="DB Camera Config" class="Bool (strict)"("Strings [4]"=w397) -> ()  [unwired: 2 in, 2 out]
      }
      event "Motor.Enable": Value Change {
        n240 = event-data() -> ("NewVal"=w405:bool)  [unwired: 1 in]
        n241 = Unbundle("Motor") -> ("Value"=w404:dbl)  [unwired: 1 out]
        n242 = Select(t=w404, s=w405, f=0.0) -> (s? t:f=w402:dbl)
        n243 = call <vilib>:"NT Write Number.vi"("Numeric"=w402, "Name"=w401) -> ()  [unwired: 9 in, 1 out]
      }
      event "Test Slider": Value Change {
        n244 = event-data() -> ("NewVal"=w408:dbl)  [unwired: 1 in]
        n245 = call <vilib>:"NT Write Number.vi"("Numeric"=w408, "Name"=w409) -> ()  [unwired: 9 in, 1 out]
      }
      event "On/Off": Value Change {
        n246 = event-data() -> ("NewVal"=w413:bool)  [unwired: 1 in]
        n247 = Boolean To (0,1)(Boolean=w413) -> (0, 1=w412:i16)
        n248 = call <vilib>:"NT Write Number.vi"("Numeric"=w412, "Name"=w411) -> ()  [unwired: 9 in, 1 out]
      }
      event "Rev/Fwd": Value Change {
        n249 = event-data() -> ("NewVal.Forward"=w421:bool, "NewVal.Reverse"=w420:bool)  [unwired: 1 in]
        n250 = Boolean To (0,1)(Boolean=w421) -> (0, 1=w417:i16)
        n251 = Boolean To (0,1)(Boolean=w420) -> (0, 1=w419:i16)
        n252 = Negate(x=w419) -> (-x=w418:i16)
        n253 = Add(x=w417, y=w418) -> (x+y=w416:i16)
        n254 = call <vilib>:"NT Write Number.vi"("Numeric"=w416, "Name"=w415) -> ()  [unwired: 9 in, 1 out]
      }
      event "Test Ring": Value Change {
        n255 = event-data() -> ("NewVal"=w425:u16)  [unwired: 1 in]
        n256 = property on="Test Ring" class="Ring (strict)"() -> ("Strings []"=w426:string[])  [unwired: 2 in, 2 out]
        n257 = Index Array(array=w426, index=w425) -> (element=w424:string)
        n258 = call <vilib>:"NT Write String.vi"("String"=w424, "Name"=w423) -> ()  [unwired: 9 in, 1 out]
      }
      event "Rec Mode": Value Change {
        # "Update globals for recording mode and path to read log from.\nClear when logging and let NetworkTables set path for vision to\nuse."
        n259 = event-data() -> ("NewVal"=w436:enum32{"Stop", "Record", "Playback"})  [unwired: 1 in]
        n260 = global write "WPI_DashboardLogging Global.vi" "Logging Filename"(path "") -> ()
        n261 = case shown="\"Playback\"" w436 {
          tunnel: w435 -> [_ w438 w446]
          tunnel: [_ _ w445] -> w432
          tunnel: [_ _ w444] -> _
          tunnel: w430 -> [_ _ w442]
          tunnel: cluster{i32, i32} {-250, 170} -> [_ _ w441]
          tunnel: [_ _ T17 {"Image Size"=TRUE, "Image Type"=TRUE, "Pixel Value"=TRUE, "ROI Information"=TRUE, "Zoom Factor"=FALSE} ("Image Information Shown:All Elements")] -> w428
          tunnel: [_ _ TRUE ("Zoom Factor")] -> w427
          frame Default {
          }
          frame "Stop", "Record" {
            # "Place Window too"
            n262 = invoke class="VI" method="FP.Close"(reference=w438) -> (reference out=w437:refnum<vi>)  [unwired: 2 in, 2 out]
            n263 = invoke class="VI" method="Abort VI"(reference=w437) -> ()  [unwired: 2 in, 3 out]
          }
          frame "Playback" {
            n264 = call "Open Playback Panel.vi"("Offset"=w441, "DB VI Ref"=w442, "Playback in"=w446) -> ("Playback out"=w443:refnum<vi>)  [unwired: 8 in]
            n265 = register-events(w443) -> (reference out=w445:refnum<event-registration>, error out=w444:errorcluster)  [unwired: 2 in]
          }
        }
        n266 = global write "WPI_DashboardLogging Global.vi" "Recording"(w436) -> ()
        n267 = property on="Camera Image" class="ImageControl"("Image Information Shown"=w428, "Image Information Visible"=w427) -> ()  [unwired: 2 in, 2 out]
        n268 = call <vilib>:"WPI_DashboardNT Log FieldName Cache.vi"("Operation"=enum16{"Lookup/Add", "Index", "Clear"}."Clear") -> ()  [unwired: 8 in, 3 out]
      }
      event Panel Close {
        w447 = enum32{"Stop", "Record", "Playback"}."Stop" ("Rec Mode")
        n269 = event-data() -> ()  [unwired: 1 in, 4 out]
        n270 = local write "Rec Mode"(w447) -> ()
        n271 = global write "WPI_DashboardLogging Global.vi" "Recording"(w447) -> ()
      }
      event Panel Close {
        # "Abort playback window and ourself"
        n272 = event-data() -> ()  [unwired: 1 in, 4 out]
        n273 = invoke class="VI" method="FP.Close"(reference=w452) -> (reference out=w451:refnum<vi>)  [unwired: 2 in, 2 out]
        n274 = invoke class="VI" method="Abort VI"(reference=w451) -> (error out=w450:errorcluster)  [unwired: 2 in, 2 out]
        n275 = invoke class="VI" method="Abort VI"(error in=w450) -> ()  [unwired: 2 in, 3 out]
      }
    }
  }
  n276 = property on="On/Off" class="Bool (strict)"("Visible"=w32) -> ()  [unwired: 2 in, 2 out]
  n277 = property on="Motor" class="Clust (strict)"("Visible"=w32) -> ()  [unwired: 2 in, 2 out]
  n278 = property on="Progress" class="Clust (strict)"("Visible"=w32) -> ()  [unwired: 2 in, 2 out]
  n279 = property on="Test Ring" class="Ring (strict)"("Visible"=w32) -> ()  [unwired: 2 in, 2 out]
  n280 = property on="Rev/Fwd" class="Clust (strict)"("Visible"=w32) -> ()  [unwired: 2 in, 2 out]
  n281 = property on="Camera Settings" class="Clust (strict)"("Visible"=w32) -> ()  [unwired: 2 in, 2 out]
  n282 = local write "DB Camera Config"(w32) -> ()
  n283 = global write "WPI_DashboardLogging Global.vi" "Recording"(w15) -> ()
  n284 = local write "Rec Mode"(w15) -> ()
  n285 = call <vilib>:"Dflt Data Dir.vi"() -> ("App:Default Data Directory"=w5:path)
  n286 = Build Path(base path=w5, name or relative path="ThresholdsCompressed.txt") -> (appended path=w2:path)
  n287 = call <vilib>:"Check if File or Folder Exists.vi"("path"=w2) -> ("file or folder exists?"=w6:bool, "dup path"=w3:path)  [unwired: 8 in, 1 out]
  n288 = case shown="False" w6 {
    tunnel: T8 [{"Blue or Luma or Val or Inten Range"={"Lower value"=0, "Upper value"=255}, "Red or Hue Range"={"Lower value"=0, "Upper value"=255}, "Green or Sat Range"={"Lower value"=0, "Upper value"=255}}, {"Blue or Luma or Val or Inten Range"={"Lower value"=0, "Upper value"=255}, "Red or Hue Range"={"Lower value"=0, "Upper value"=255}, "Green or Sat Range"={"Lower value"=0, "Upper value"=255}}, {"Blue or Luma or Val or Inten Range"={"Lower value"=0, "Upper value"=255}, "Red or Hue Range"={"Lower value"=0, "Upper value"=255}, "Green or Sat Range"={"Lower value"=0, "Upper value"=255}}] ("Threshold Values") -> [w453 w457]
    tunnel: w3 -> [_ w456]
    tunnel: [w453 w454] -> w1
    frame False {
    }
    frame True {
      n289 = Read from Text File(file (use dialog)=w456) -> (text=w455:string)  [unwired: 3 in, 3 out]
      n290 = Unflatten From String(type=w457, binary string=w455) -> (value=w454:T8)  [unwired: 3 in, 2 out]
    }
  }
  n291 = while {
    tunnel: w2 -> [w458]
    stop <- FALSE stop-if-true
    n292 = flat-sequence {
      tunnel: w458 -> [w462]
      frame #0 {
        n293 = Wait (ms)(milliseconds to wait=1000) -> ()  [unwired: 1 out]
      }
      frame #1 {
        n294 = local read "Threshold Values"() -> (w463:T8)
        n295 = Flatten To String(anything=w463) -> (data string=w464:string, error out=w461:errorcluster)  [unwired: 3 in, 1 out]
        n296 = Write to Text File(file (use dialog)=w462, text=w464, error in=w461) -> ()  [unwired: 1 in, 3 out]
      }
    }
  }
  n297 = local write "Threshold Values"(w1) -> ()
